vi "VoltageSetting.vi"(11 "Cohort Setting":i8[](array[numeric])) -> (3 "Voltages":sgl[](array[numeric]))   [LabVIEW 2012]
uses:
  AmplitudePanel.ctl
  CohortPanel.ctl
  StimulCtrls.lvlib
panel:
  in  "Electrode Panel":T1={"0"=2, "1"=0, "2"=0, "3"=0, "4"=0, "5"=2, "6"=1, "7"=0, "8"=0, "9"=0, "10"=0, "11"=2, "12"=0, "13"=0, "14"=0, "15"=0}
  out "error out":errorcluster
  in  "OK Button":bool
  in  "Voltage Control":T2={"0"=2, "1"=2, "2"=2, "3"=2, "4"=2, "5"=2, "6"=2, "7"=2, "8"=2, "9"=2, "10"=2, "11"=2, "12"=2, "13"=2, "14"=2, "15"=2} {"15" scale=0.0..10.0; "14" scale=0.0..10.0; "13" scale=0.0..10.0; "12" scale=0.0..10.0; "11" scale=0.0..10.0; "10" scale=0.0..10.0; "9" scale=0.0..10.0; "8" scale=0.0..10.0; "7" scale=0.0..10.0; "6" scale=0.0..10.0; "5" scale=0.0..10.0; "4" scale=0.0..10.0; "3" scale=0.0..10.0; "2" scale=0.0..10.0; "1" scale=0.0..10.0; "0" scale=0.0..10.0}
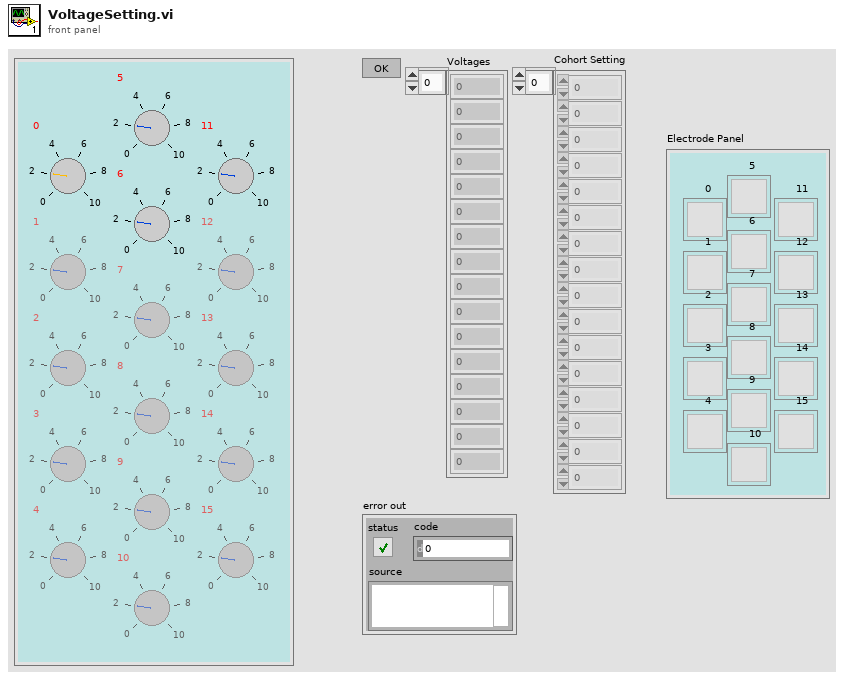
[diagram p1: front panel]
types:
  T1 = typedef "StimulCtrls.lvlib/CohortPanel.ctl" = cluster{"0":u16, "1":u16, "2":u16, "3":u16, "4":u16, "5":u16, "6":u16, "7":u16, "8":u16, "9":u16, "10":u16, "11":u16, "12":u16, "13":u16, "14":u16, "15":u16}
  T2 = typedef "StimulCtrls.lvlib/AmplitudePanel.ctl" = cluster{"0":u16, "1":u16, "2":u16, "3":u16, "4":u16, "5":u16, "6":u16, "7":u16, "8":u16, "9":u16, "10":u16, "11":u16, "12":u16, "13":u16, "14":u16, "15":u16}
  T3 = enum32{"Invalid", "Standard", "Closed", "Hidden", "Minimized", "Maximized"}
  T4 = cluster{"[0]":i32, "[1]":i32, "[2]":i32, "[3]":i32, "[4]":i32, "[5]":i32, "[6]":i32, "[7]":i32, "[8]":i32, "[9]":i32, "[10]":i32, "[11]":i32, "[12]":i32, "[13]":i32, "[14]":i32, "[15]":i32}
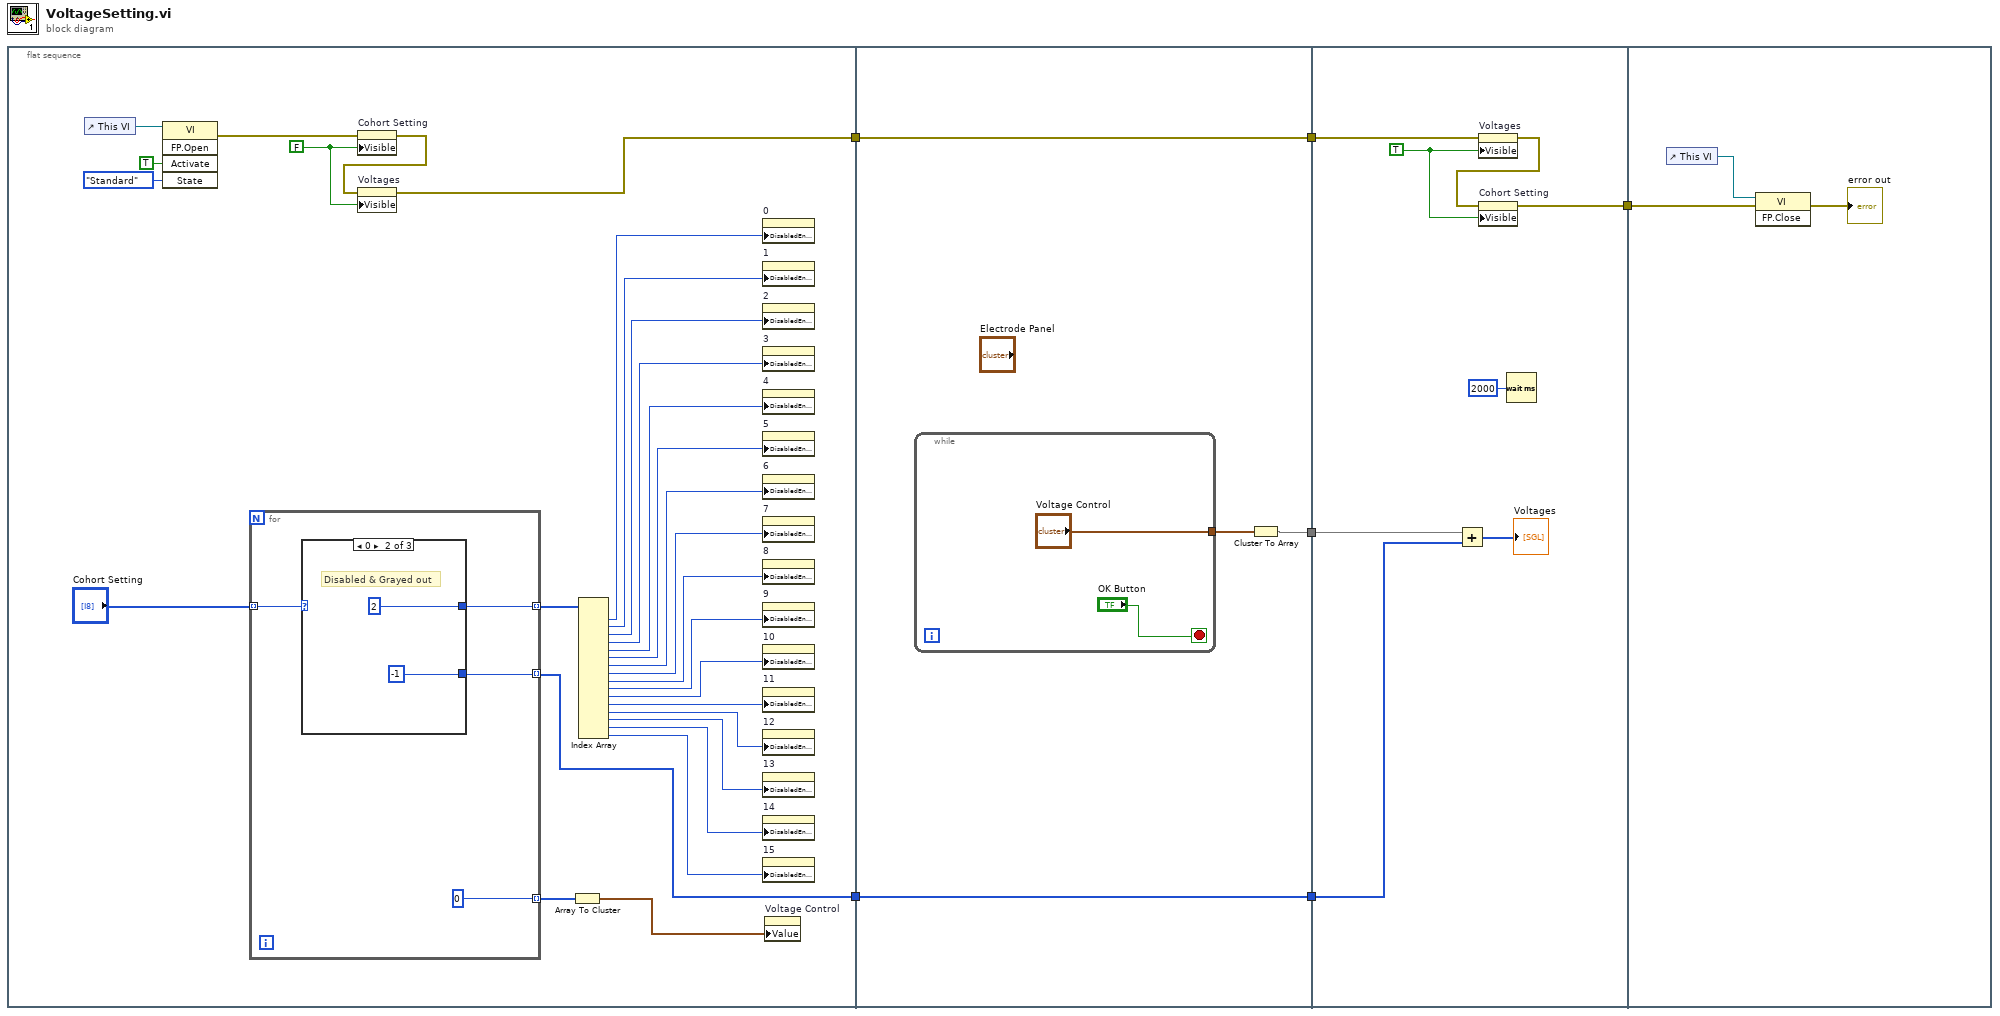
[diagram p0: block diagram]
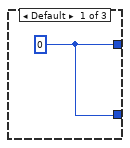
[diagram p2: hidden frame]
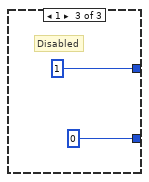
[diagram p3: hidden frame]
diagram:
  n1 = flat-sequence {
    tunnel: [w14] -> w6
    tunnel: [w11] -> w2
    tunnel: w6 -> [w47]
    tunnel: [w47] -> w5
    tunnel: [w45] -> w4
    tunnel: [w44] -> w3
    tunnel: w2 -> [w44]
    tunnel: w5 -> [w54]
    tunnel: w4 -> [w55]
    tunnel: w3 -> [w52]
    tunnel: [w50] -> w1
    tunnel: w1 -> [w59]
    frame #0 {
      w13 = FALSE
      n2 = control-ref of="This VI"() -> (w10:refnum<vi>)
      n3 = invoke class="VI" method="FP.Open"(reference=w10, "Activate"=TRUE ("Activate?"), "State"=T3."Standard") -> (error out=w7:errorcluster)  [unwired: 2 in, 4 out]
      n4 = for {
        tunnel: "Cohort Setting" -> [w37] mode=indexing
        tunnel: [w38] -> w32 mode=indexing
        tunnel: [0] -> w16 mode=indexing
        tunnel: [w35] -> w14 mode=indexing
        n5 = case shown="0" w37 {
          tunnel: [w39 2 1] -> w38
          tunnel: [w39 -1 0] -> w35
          frame Default {
            w39 = 0
          }
          frame 0 {
            # "Disabled & Grayed out"
          }
          frame 1 {
            # "Disabled"
          }
        }
      }
      n6 = property on="Cohort Setting" class="Arr (strict)"(error in=w7, "Visible"=w13) -> (error out=w12:errorcluster)  [unwired: 1 in, 1 out]
      n7 = property on="Voltages" class="Arr (strict)"(error in=w12, "Visible"=w13) -> (error out=w11:errorcluster)  [unwired: 1 in, 1 out]
      n8 = Array To Cluster(array=w16) -> (cluster=w15:T4)
      n9 = Index Array(array=w32) -> (element #1=w33:i32, element #2=w31:i32, element #3=w30:i32, element #4=w29:i32, element #5=w28:i32, element #6=w27:i32, element #7=w26:i32, element #8=w25:i32, element #9=w24:i32, element #10=w23:i32, element #11=w22:i32, element #12=w21:i32, element #13=w20:i32, element #14=w19:i32, element #15=w18:i32, element #16=w17:i32)  [unwired: 16 in]
      n10 = property on="0" class="Knob (strict)"("DisabledEnum"=w33) -> ()  [unwired: 2 in, 2 out]
      n11 = property on="1" class="Knob (strict)"("DisabledEnum"=w31) -> ()  [unwired: 2 in, 2 out]
      n12 = property on="2" class="Knob (strict)"("DisabledEnum"=w30) -> ()  [unwired: 2 in, 2 out]
      n13 = property on="3" class="Knob (strict)"("DisabledEnum"=w29) -> ()  [unwired: 2 in, 2 out]
      n14 = property on="4" class="Knob (strict)"("DisabledEnum"=w28) -> ()  [unwired: 2 in, 2 out]
      n15 = property on="5" class="Knob (strict)"("DisabledEnum"=w27) -> ()  [unwired: 2 in, 2 out]
      n16 = property on="6" class="Knob (strict)"("DisabledEnum"=w26) -> ()  [unwired: 2 in, 2 out]
      n17 = property on="7" class="Knob (strict)"("DisabledEnum"=w25) -> ()  [unwired: 2 in, 2 out]
      n18 = property on="8" class="Knob (strict)"("DisabledEnum"=w24) -> ()  [unwired: 2 in, 2 out]
      n19 = property on="9" class="Knob (strict)"("DisabledEnum"=w23) -> ()  [unwired: 2 in, 2 out]
      n20 = property on="10" class="Knob (strict)"("DisabledEnum"=w22) -> ()  [unwired: 2 in, 2 out]
      n21 = property on="11" class="Knob (strict)"("DisabledEnum"=w21) -> ()  [unwired: 2 in, 2 out]
      n22 = property on="12" class="Knob (strict)"("DisabledEnum"=w20) -> ()  [unwired: 2 in, 2 out]
      n23 = property on="13" class="Knob (strict)"("DisabledEnum"=w19) -> ()  [unwired: 2 in, 2 out]
      n24 = property on="14" class="Knob (strict)"("DisabledEnum"=w18) -> ()  [unwired: 2 in, 2 out]
      n25 = property on="15" class="Knob (strict)"("DisabledEnum"=w17) -> ()  [unwired: 2 in, 2 out]
      n26 = property on="Voltage Control" class="Clust (strict)"("Value"=w15) -> ()  [unwired: 2 in, 2 out]
    }
    frame #1 {
      n27 = while {
        tunnel: ["Voltage Control"] -> w46
        stop <- "OK Button" stop-if-true
      }
      n28 = Cluster To Array(cluster=w46) -> (array=w45:u16[])
    }
    frame #2 {
      w57 = TRUE
      n29 = Add(x=w55, y=w54) -> (x+y=→"Voltages":i32[])
      n30 = property on="Voltages" class="Arr (strict)"(error in=w52, "Visible"=w57) -> (error out=w53:errorcluster)  [unwired: 1 in, 1 out]
      n31 = property on="Cohort Setting" class="Arr (strict)"(error in=w53, "Visible"=w57) -> (error out=w50:errorcluster)  [unwired: 1 in, 1 out]
      n32 = Wait (ms)(milliseconds to wait=u32 2000) -> ()  [unwired: 1 out]
    }
    frame #3 {
      n33 = control-ref of="This VI"() -> (w60:refnum<vi>)
      n34 = invoke on="Invoke Node" class="VI" method="FP.Close"(reference=w60, error in=w59) -> (error out=→"error out":errorcluster)  [unwired: 1 in, 2 out]
    }
  }
